vi "FRCts20_WebMethods_BackendError.vi"(7 "Prev Status":string="Success", 8 "error in (no error)":errorcluster, 10 "Status":string) -> (0 "error out":errorcluster, 2 "Status out":string)   [LabVIEW 2013, in "FRCts20_WebMethods.lvlib"]
doc: "Interprets the <B>Status</B> output of the Backend API.\n\nIf a fatal or unknown error was returned, the error is injected into the error wire. Status messages indicating incorrect HTTP requests are interpreted and output on <B>Status out</B> (no error is returned).\n\n<B>Status out -</B> \"Backend Error\": Fatal or unexpected error\n \"No Action\": Resource already/does not exist\n \"Success\": Request successfully processed"
uses:
  FRCts20_WebMethods.lvlib
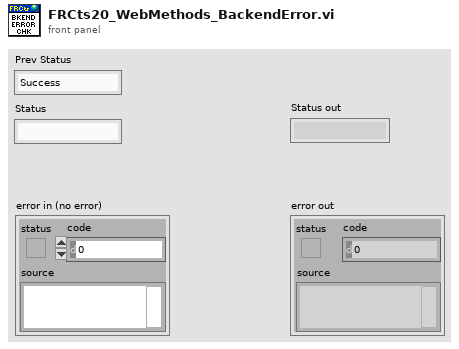
[diagram p1: front panel]
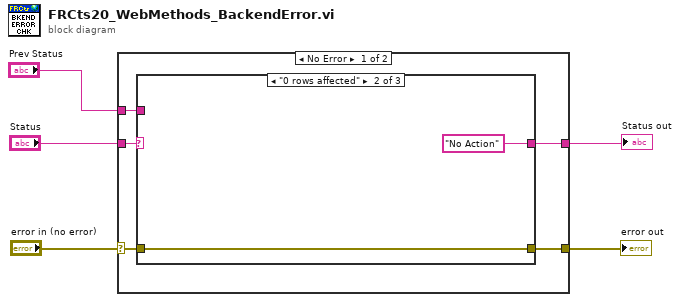
[diagram p0: block diagram]
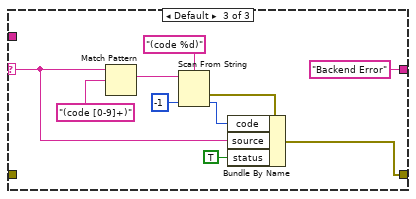
[diagram p3: hidden frame]
diagram:
  n1 = case shown="No Error" "error in (no error)" {
    selector: "error in (no error)" -> [w8 w25]
    tunnel: "Status" -> [w10 w26]
    tunnel: [w9 w26] -> w2
    tunnel: [w7 w25] -> w3
    tunnel: "Prev Status" -> [w6 _]
    frame No Error {
      n2 = case shown="\"0 rows affected\"" w10 {
        selector: w10 -> [_ _ w20]
        tunnel: [w11 "No Action" "Backend Error"] -> w9
        tunnel: w8 -> [w12 w13 _]
        tunnel: [w12 w13 w21] -> w7
        tunnel: w6 -> [w11 _ _]
        frame "Success" {
        }
        frame "0 rows affected" {
        }
        frame Default {
          n3 = Match Pattern(string=w20, regular expression="(code [0-9]+)") -> (match substring=w18:string)  [unwired: 1 in, 3 out]
          n4 = Scan From String(format string="(code %d)", input string=w18, default 1=-1 ("default value 1")) -> (error out=w15:errorcluster, output 1=w16:i32)  [unwired: 2 in, 2 out]
          n5 = Bundle By Name(cluster=w15, "code"=w16, "source"=w20, "status"=TRUE) -> (w21:errorcluster)
        }
      }
    }
    frame Error {
    }
  }
  "error out" <- w3
  "Status out" <- w2
